vi "get_amplitude.vi"(8 "error in (no error)":errorcluster, 11 "Function Generator in":refnum<class "Function Generator.lvclass">) -> (0 "error out":errorcluster, 2 "Amplitude":dbl, 3 "Function Generator out":refnum<class "Function Generator.lvclass">)   [LabVIEW 2020, in "Function Generator.lvclass"]
uses:
  Function Generator.lvclass
  Function Generator.lvclass/Function Generator.ctl
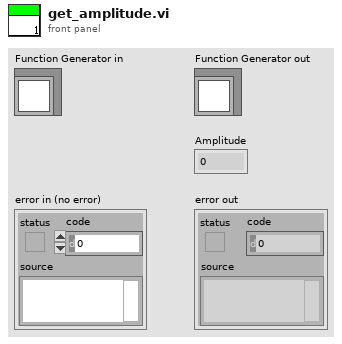
[diagram p1: front panel]
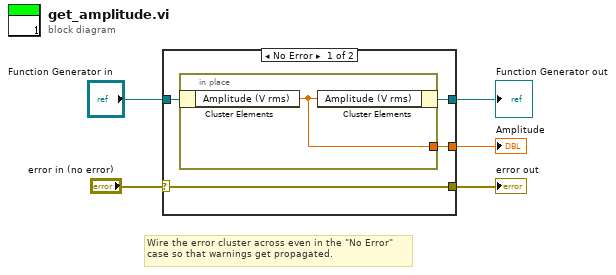
[diagram p0: block diagram]
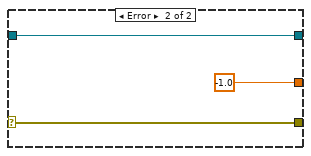
[diagram p2: hidden frame]
diagram:
  # "Wire the error cluster across even in the \"No Error\"\ncase so that warnings get propagated."
  n1 = case shown="No Error" "error in (no error)" {
    selector: "error in (no error)" -> [w9 w13]
    tunnel: [w9 w13] -> w4
    tunnel: [w7 w12] -> w2
    tunnel: "Function Generator in" -> [w8 w12]
    tunnel: [w6 -1.0] -> w1
    frame No Error {
      n2 = in-place {
        in-place-border: [w10] -> w6
        n3 = in-place-cluster #1(w8) -> ("Amplitude (V rms)"=w10:dbl)
        n4 = in-place-cluster #1("Amplitude (V rms)"=w10) -> (w7:refnum<class "Function Generator.lvclass">)
      }
    }
    frame Error {
    }
  }
  "error out" <- w4
  "Function Generator out" <- w2
  "Amplitude" <- w1
